vi "GetPressure.vi"(8 "error in (no error)":errorcluster, 11 "MKS901P in":refnum<class "MKS901P.lvclass">) -> (0 "error out":errorcluster, 2 "Pressure (mbar)":dbl, 3 "MKS901P out":refnum<class "MKS901P.lvclass">)   [LabVIEW 2016, in "MKS901P.lvlib" / "MKS901P.lvclass"]
uses:
  MKS901P.lvclass
  MKS901P.lvclass/MKS901P.ctl
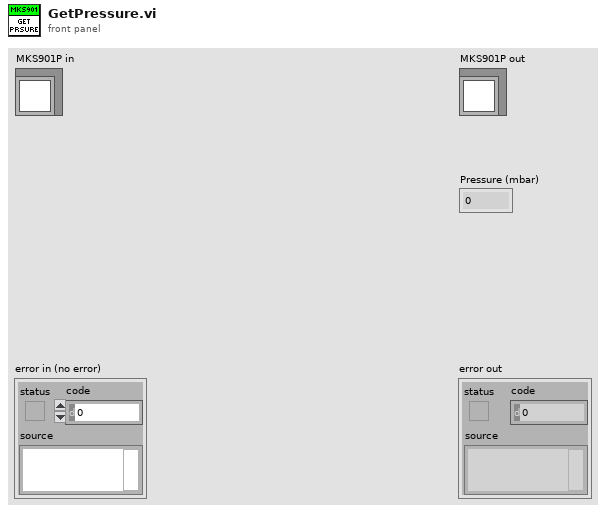
[diagram p1: front panel]
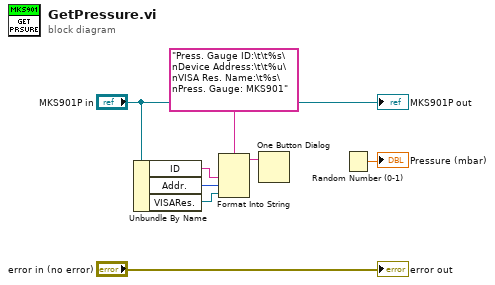
[diagram p0: block diagram]
diagram:
  n1 = Unbundle By Name("MKS901P in") -> ("ID"=w6:string, "Addr."=w7:u8, "VISARes."=w5:refnum<visa-resource-name>)
  n2 = Format Into String(format string="Press. Gauge ID:\t\t%s\nDevice Address:\t\t%u\nVISA Res. Name:\t%s\nPress. Gauge: MKS901", w6, w7, w5) -> (resulting string=w4:string)  [unwired: 2 in, 1 out]
  n3 = One Button Dialog(message=w4) -> ()  [unwired: 1 in, 1 out]
  n4 = Random Number (0-1)() -> (number: 0 to 1=→"Pressure (mbar)":dbl)
  "error out" <- "error in (no error)"
  "MKS901P out" <- "MKS901P in"
